vi "Mutex Attr Get Mutex Type.vi"(8 "error in (no error)":errorcluster, 11 "Mutex Attr in":T2) -> (0 "error out":errorcluster, 2 "mutex type":T1, 3 "Mutex Attr out":T2)   [LabVIEW 2016, in "Linux RT IPC.POSIX Threads.lvlib" / "Mutex Attr.lvclass"]
doc: "Calls pthread_mutexattr_gettype() on the pthread mutex attribute object encapsulated by Mutex Attr.\n\nThis VI gets the current mutex type defined in the mutex attribute object.\n\nRefer to online POSIX documentation for more information."
uses:
  Mutex Attr.lvclass
  Controls/reference.ctl
  C:/Git/SourceTree/LinuxRT-IPC/Source/POSIX Threads/Classes/POSIX Thread Object/POSIX Thread Object.lvclass
  Controls/Public/C Enums/pthread_mutex_type.ctl
  POSIX Thread Object/POSIX Thread Object.lvclass/POSIX Thread Object.ctl
  POSIX Thread Object/Private VIs/libpthread path.vi
  POSIX Thread Object/Private VIs/get pthread error.vi
  POSIX Thread Object/POSIX Thread Object.lvclass
  Linux RT IPC.POSIX Threads.lvlib
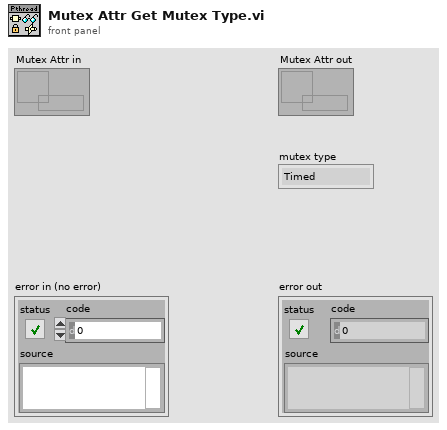
[diagram p1: front panel]
types:
  T1 = typedef "Linux RT IPC.POSIX Threads.lvlib/pthread_mutex_type.ctl" = enum16{"Timed", "Recursive", "Errorcheck", "Adaptive"}
  T2 = typedef "Linux RT IPC.POSIX Threads.lvlib/Mutex Attr.lvclass/reference.ctl" = refnum<data-value>
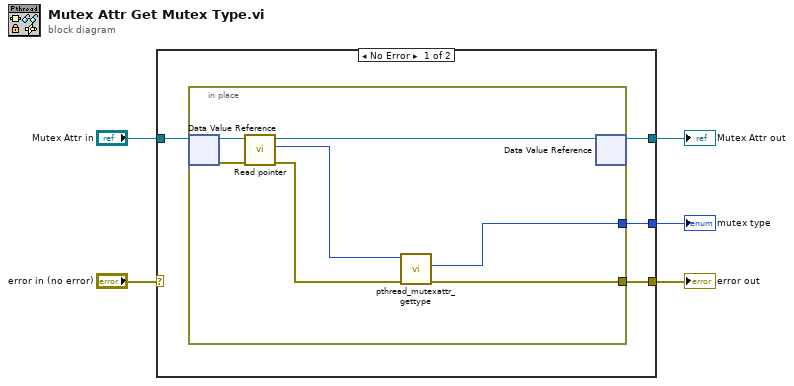
[diagram p0: block diagram]
diagram:
  n1 = case shown="No Error" "error in (no error)" {
    selector: "error in (no error)" -> [_ w18]
    tunnel: [w7 w18] -> w4
    tunnel: "Mutex Attr in" -> [w9 w17]
    tunnel: [w8 w17] -> w2
    tunnel: [w6 _] -> w1
    frame No Error {
      n2 = in-place {
        in-place-border: [w12] -> w7
        in-place-border: [w10] -> w6
        n3 = in-place-dvr #1(w9) -> (w16:refnum<class "Mutex Attr.lvclass">, w14:errorcluster)
        n4 = call "Read pointer.vi"("error in (no error)"=w14, "POSIX Thread Object in"=w16) -> ("error out"=w13:errorcluster, "pointer"=w11:u64, "POSIX Thread Object out"=w15:refnum<class "Mutex Attr.lvclass">)  [unwired: 7 in]
        n5 = call "pthread_mutexattr_gettype.vi"("error in (no error)"=w13, "mutex attr ptr in"=w11) -> ("error out"=w12:errorcluster, "mutex type"=w10:T1)  [unwired: 7 in, 1 out]
        n6 = in-place-dvr #1(w15) -> (w8:T2)  [unwired: 1 out]
      }
    }
    frame Error {
    }
  }
  "Mutex Attr out" <- w2
  "error out" <- w4
  "mutex type" <- w1
